vi "Dispose.vi"(8 "error in (no error)":errorcluster caption="错误输入（无错误）", 11 "Mediator 输入":refnum<class "Mediator.lvclass"> caption="DNL_LabVIEW Object in") -> (0 "error out":errorcluster caption="错误输出", 3 "Mediator 输出":refnum<class "Mediator.lvclass"> caption="DNL_LabVIEW Object out")   [LabVIEW 2011, in "Mediator.lvclass"]
uses:
  Mediator.lvclass
  Mediator.lvclass/Mediator.ctl
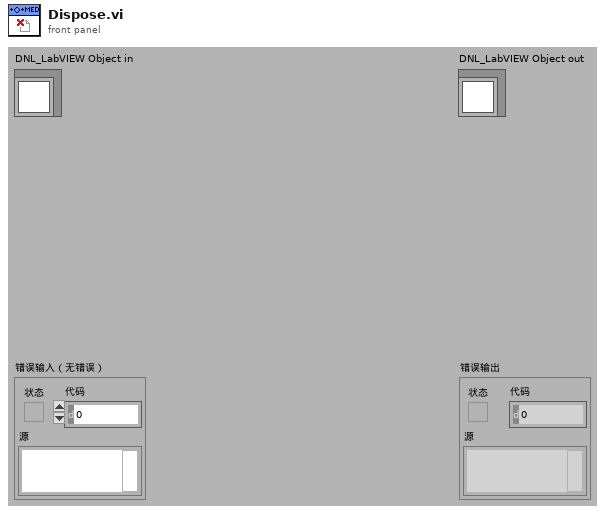
[diagram p1: front panel]
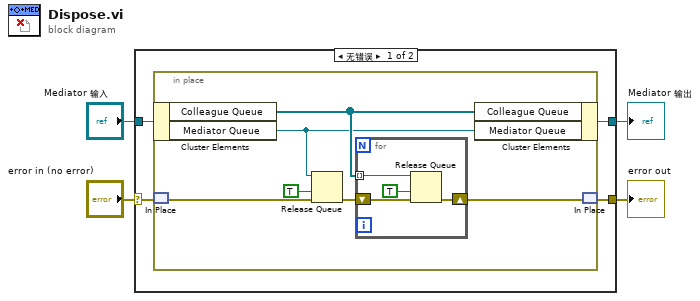
[diagram p0: block diagram]
diagram:
  n1 = case shown="无错误" "error in (no error)" {
    selector: "error in (no error)" -> [w7 w20]
    tunnel: [w6 w20] -> w3
    tunnel: [w5 w19] -> w1
    tunnel: "Mediator 输入" -> [w8 w19]
    frame No Error {
      n2 = in-place {
        n3 = in-place-cluster #1(w8) -> ("Colleague Queue"=w11:refnum<queue>[], "Mediator Queue"=w10:refnum<queue>)
        n4 = in-place-match #2(w7) -> (w14:errorcluster)
        n5 = Release Queue(queue=w10, force destroy? (F)=TRUE ("强制销毁？(F)"), error in (no error)=w14) -> (error out=w12:errorcluster)  [unwired: 2 out]
        n6 = for {
          shift-right: [w18] -> w9
          shift-left: w12 -> [w16]
          tunnel: w11 -> [w15] mode=indexing
          n7 = Release Queue(queue=w15, force destroy? (F)=TRUE ("强制销毁？(F)"), error in (no error)=w16) -> (error out=w18:errorcluster)  [unwired: 2 out]
        }
        n8 = in-place-cluster #1("Colleague Queue"=w11, "Mediator Queue"=w10) -> (w5:refnum<class "Mediator.lvclass">)
        n9 = in-place-match #2(w9) -> (w6:errorcluster)
      }
    }
    frame Error {
    }
  }
  "error out" <- w3
  "Mediator 输出" <- w1
